vi "UDLR (ASCII Arrows).vi"() -> (3 "UDLR (ASCII Arrows)":u8[](array[numeric]))   [LabVIEW 2025, in "AOC.lvlib"]
uses:
  AOC.lvlib
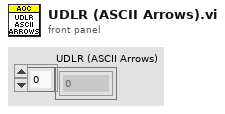
[diagram p1: front panel]
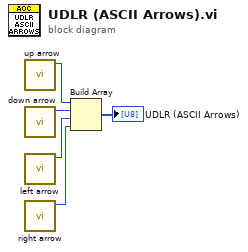
[diagram p0: block diagram]
diagram:
  n1 = call "up arrow.vi"() -> ("^"=w1:u8)  [unwired: 11 in]
  n2 = call "down arrow.vi"() -> ("v"=w2:u8)  [unwired: 11 in]
  n3 = call "left arrow.vi"() -> ("<"=w3:u8)  [unwired: 11 in]
  n4 = call "right arrow.vi"() -> (">"=w4:u8)  [unwired: 11 in]
  n5 = Build Array(w1, w2, w3, w4) -> (→"UDLR (ASCII Arrows)":u8[])
